vi "Calculate Distance to run.vi"(3 "Distance to Target (ft)":dbl) -> (0 "Distance to Travel (m)":dbl, 1 "Robot move forward":bool)   [LabVIEW 2015]
uses:
  Global Variables/Calibrations.vi
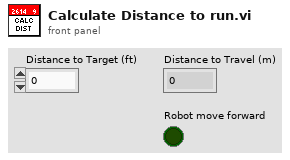
[diagram p1: front panel]
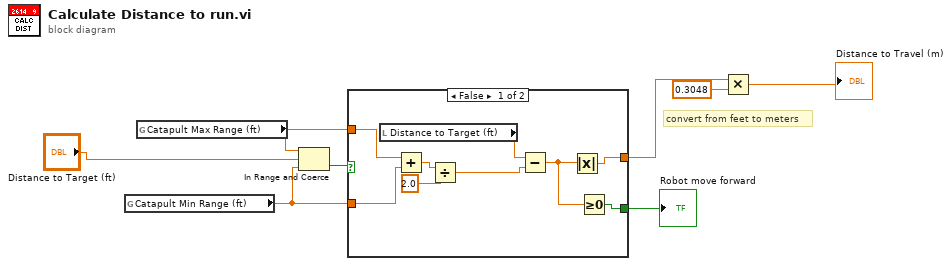
[diagram p0: block diagram]
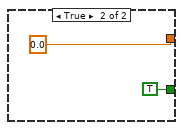
[diagram p2: hidden frame]
diagram:
  # "convert from feet to meters"
  n1 = global read "Calibrations.vi" "Catapult Min Range (ft)"() -> (w5:dbl)
  n2 = global read "Calibrations.vi" "Catapult Max Range (ft)"() -> (w6:dbl)
  n3 = In Range and Coerce(upper limit=w6, x="Distance to Target (ft)", lower limit=w5) -> (In Range?=w7:bool)  [unwired: 1 out]
  n4 = case shown="False" w7 {
    tunnel: [w12 0.0] -> w3
    tunnel: w6 -> [w17 _]
    tunnel: w5 -> [w16 _]
    tunnel: [w9 TRUE] -> w4
    frame False {
      n5 = local read "Distance to Target (ft)"() -> (w13:dbl)
      n6 = Add(x=w17, y=w16) -> (x+y=w15:dbl)
      n7 = Divide(x=w15, y=2.0) -> (x/y=w11:dbl)
      n8 = Subtract(x=w13, y=w11) -> (x-y=w10:dbl)
      n9 = Absolute Value(x=w10) -> (abs(x)=w12:dbl)
      n10 = Greater Or Equal To 0?(x=w10) -> (x >= 0?=w9:bool)
    }
    frame True {
    }
  }
  "Robot move forward" <- w4
  n11 = Multiply(x=w3, y=0.3048) -> (x*y=→"Distance to Travel (m)":dbl)
